vi "SimplePulseGenerator.vi"() -> ()   [LabVIEW 2012]
uses:
  <vilib>/Utility/sysdir.llb/System Directory Type.ctl
  <vilib>/Utility/miscctls.llb/LVPointTypeDef.ctl
  <vilib>/DAQmx/create/channels.llb/DAQmx Create Channel (CO-Pulse Generation-Frequency).vi
  <vilib>/DAQmx/configure/timing.llb/DAQmx Timing (Implicit).vi
  <resource>/objmgr/daqmx.rc
panel:
  out "title":string="Simple PulseGenerator"
  in  "Output Pulse Count":u64 caption="Pulse" format="%.0p"
  in  "Chk Finite":bool
  in  "Duty Cycle(%)":i32(slide)=50 scale=1.0..99.0
  in  "Counter Ch":tag="Dev1/ctr0"
  in  "Idle State":i32(ring)=10214 items=["High"=10192, "Low"=10214]
  in  "Frequency(Hz)":i32(knob)=1000 scale=1.0..1000000.0 scale format="%.0p"
  in  "Output":bool caption="Output Sw"
  # "with DAQmx Driver"
  # "%"
  # "Hz"
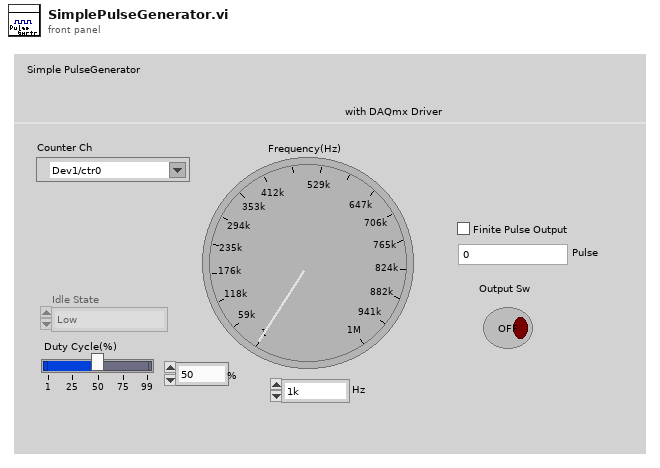
[diagram p1: front panel]
types:
  T1 = enum32{"invalid app kind", "Development System", "Run Time System", "Student Edition", "Embedded LabVIEW", "Evaluation", "Custom"}
  T2 = typedef "System Directory Type.ctl" = i32
  T3 = typedef "LVPointTypeDef.ctl" = cluster{"Horizontal":i16, "Vertical":i16}
  T4 = cluster{bool, "include Ctrl key?":bool, string}[]
  T5 = cluster{"配列[0]":i16, "配列[1]":i16, "配列[2]":i16, "配列[3]":i16}
  T6 = typedef "LVRectTypeDef.ctl" = cluster{"Left":i16, "Top":i16, "Right":i16, "Bottom":i16}
  T7 = enum8{"Enabled", "Disabled", "Disabled and Grayed Out"}
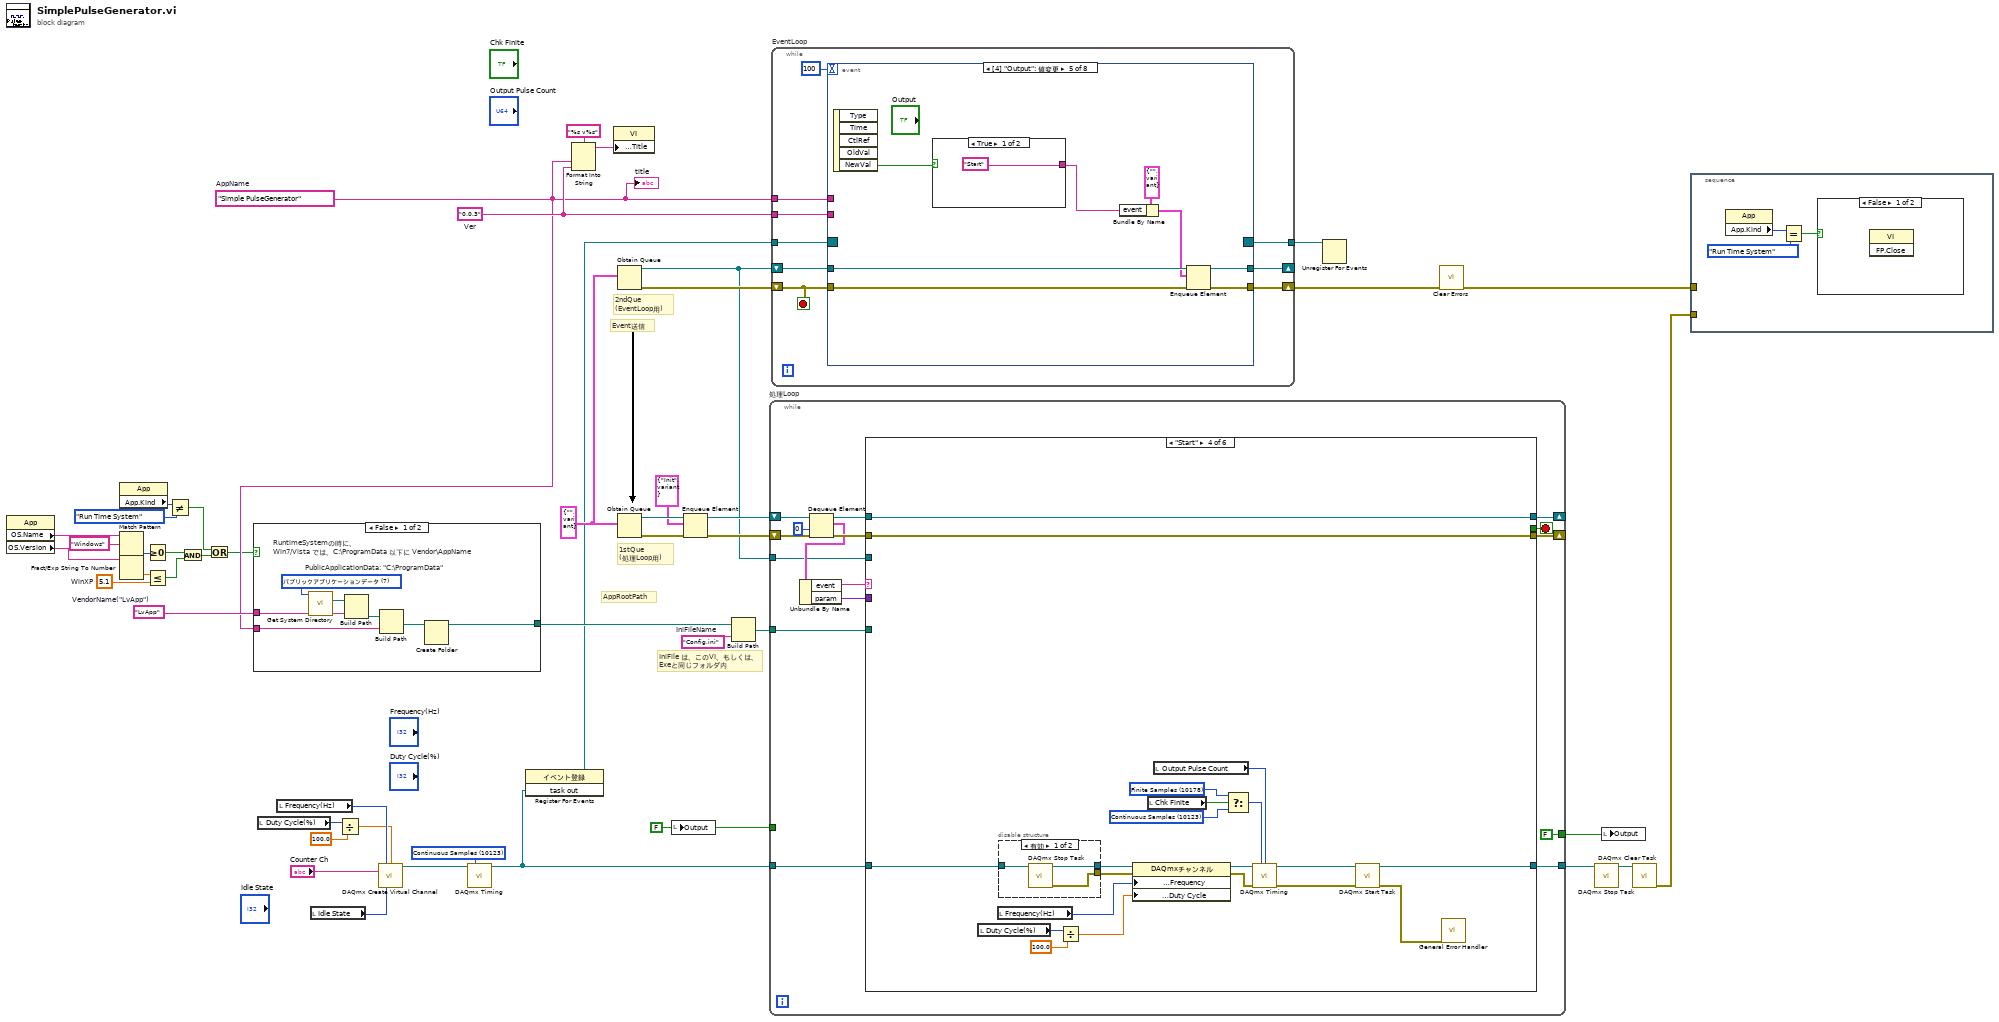
[diagram p0: block diagram]
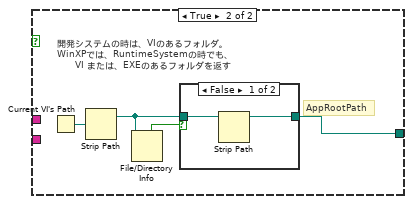
[diagram p2: hidden frame]
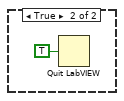
[diagram p4: hidden frame]
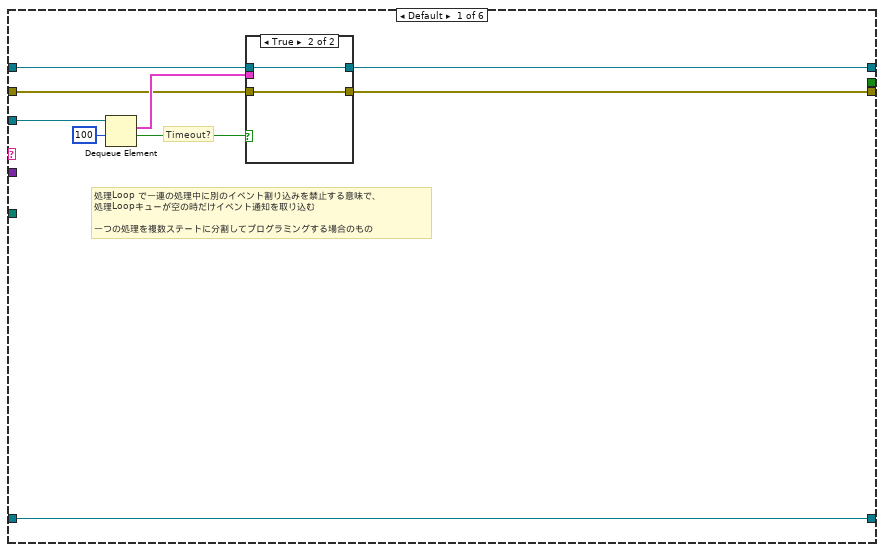
[diagram p5: hidden frame]
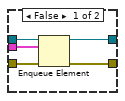
[diagram p6: hidden frame]
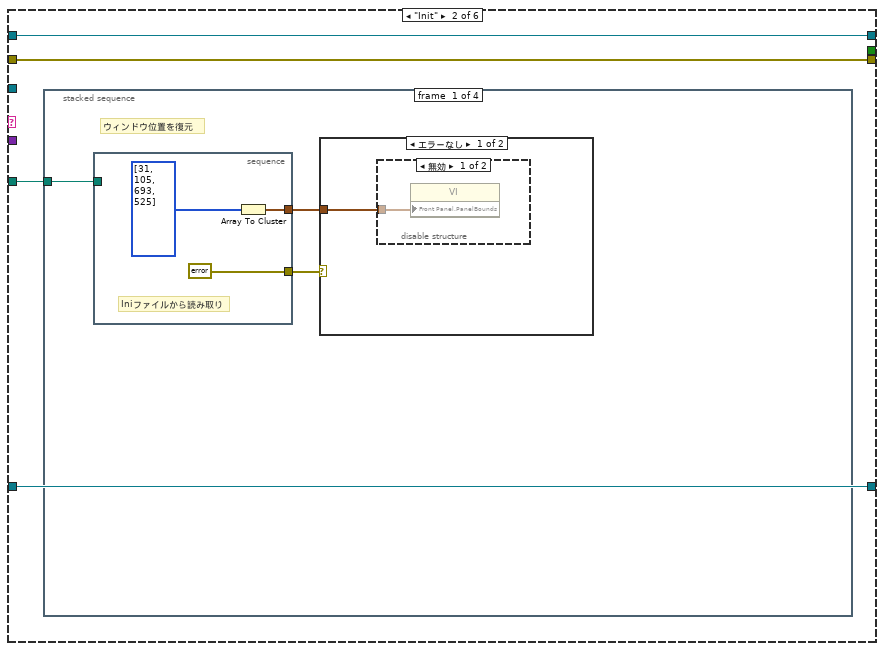
[diagram p7: hidden frame]
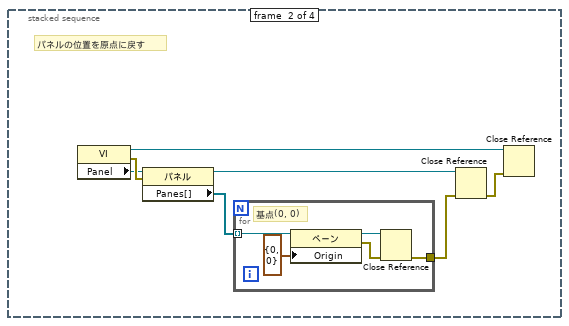
[diagram p10: hidden frame]
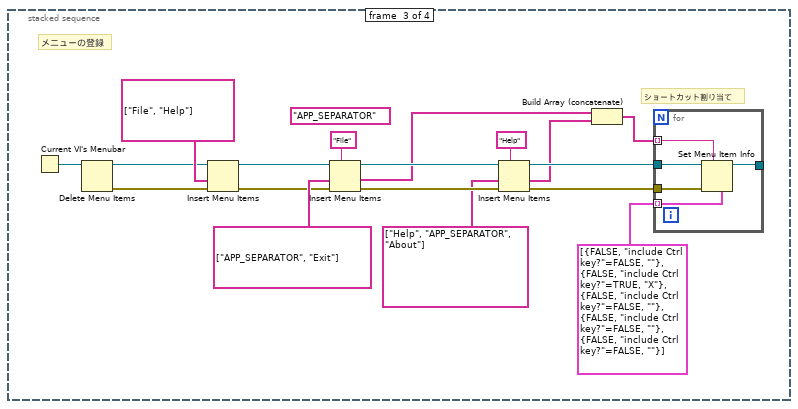
[diagram p11: hidden frame]
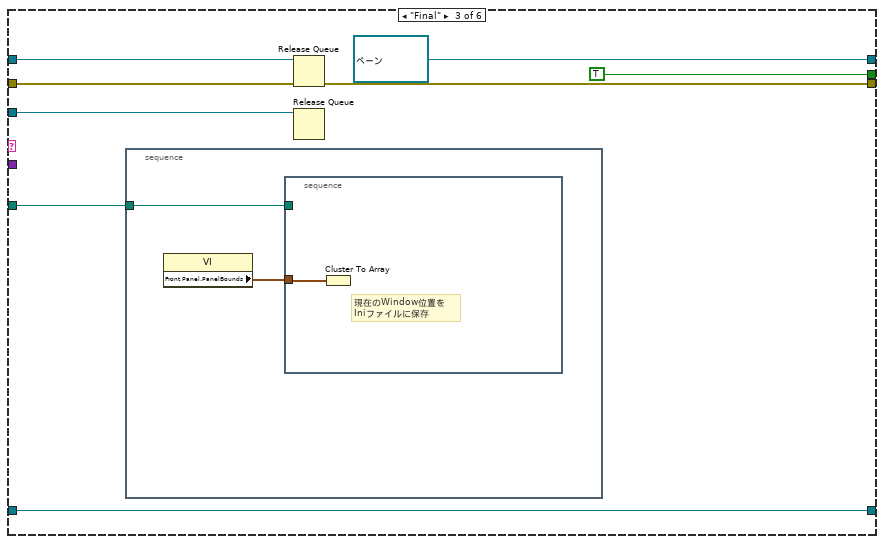
[diagram p13: hidden frame]
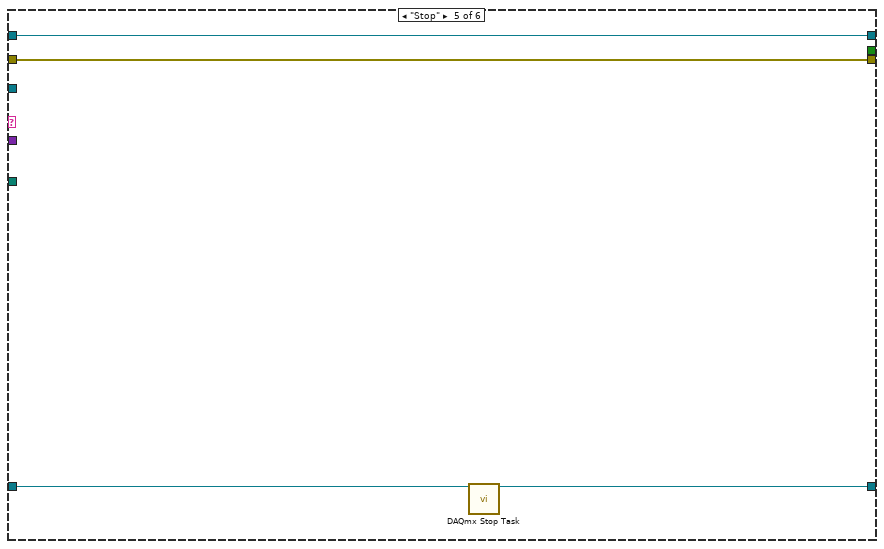
[diagram p15: hidden frame]
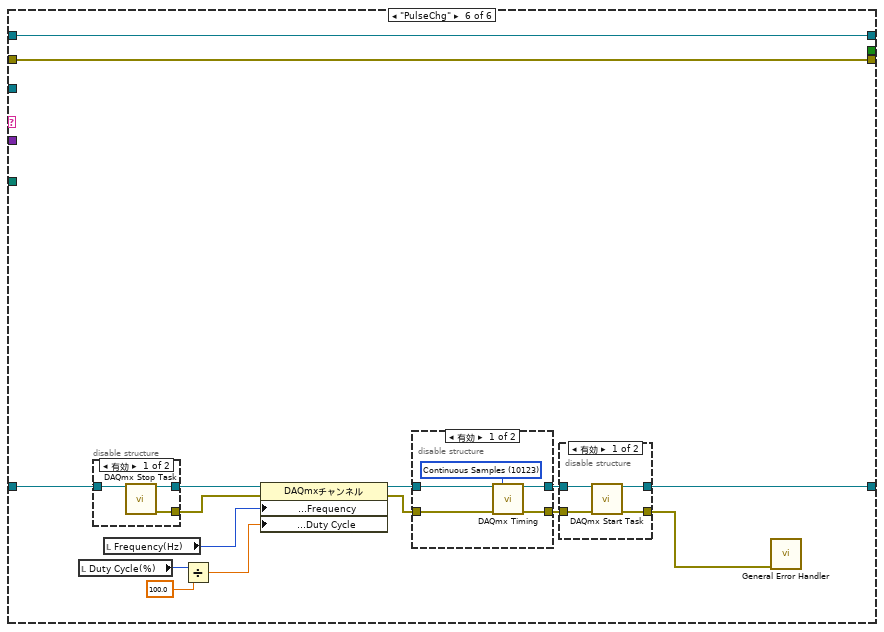
[diagram p16: hidden frame]
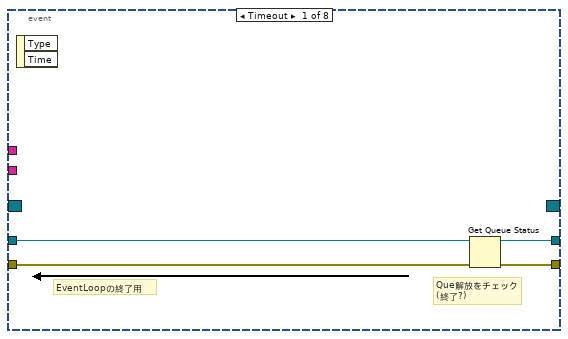
[diagram p20: hidden frame]
diagram:
  w6 = 10123 items=["Finite Samples"=10178, "Continuous Samples"=10123] ("sample mode")
  w12 = cluster{"event":string, "param":variant} {"event"="", "param"=variant}
  w14 = FALSE ("Output")
  w24 = "LvApp"  # VendorName("LvApp")
  w29 = 5.1  # WinXP
  w34 = "Config.ini"  # IniFileName
  w37 = "0.0.3"  # Ver
  w23 = "Simple PulseGenerator"  # AppName
  # "IniFile は、このVI、もしくは、\nExeと同じフォルダ内"
  # "AppRootPath"
  # "2ndQue\n(EventLoop用)"
  # "1stQue\n(処理Loop用)"
  # "Event送信"
  n1 = property class="App"() -> ("OS.Name"=w33:string, "OS.Version"=w31:string)  [unwired: 2 in, 2 out]
  n2 = Match Pattern(string=w33, regular expression="Windows" ("正規表現")) -> (offset past match=w28:i32)  [unwired: 1 in, 3 out]
  n3 = Fract/Exp String To Number(string=w31) -> (number=w30:dbl)  [unwired: 3 in, 1 out]
  n4 = property class="App"() -> ("App.Kind"=w22:T1)  [unwired: 2 in, 2 out]
  n5 = Greater Or Equal To 0?(x=w28) -> (x >= 0?=w27:bool)
  n6 = Less Or Equal?(x=w30, y=w29) -> (x <= y?=w26:bool)
  n7 = Not Equal?(x=w22, y=T1."Run Time System" ("アプリケーション:種類")) -> (x != y?=w20:bool)
  n8 = And(x=w27, y=w26) -> (x .and. y?=w19:bool)
  n9 = Or(x=w20, y=w19) -> (x .or. y?=w18:bool)
  n10 = case shown="FALSE" w18 {
    tunnel: w23 -> [w51 _]
    tunnel: [w48 w55] -> w25
    tunnel: w24 -> [w49 _]
    frame False {
      w54 = T2 7 items=["ユーザホーム"=0, "ユーザデスクトップ"=1, "ユーザドキュメント"=2, "ユーザアプリケーションデータ"=3, "ユーザ設定"=4, "ユーザ一時"=5, "パブリックドキュメント"=6, "パブリックアプリケーションデータ"=7, "パブリック環境設定"=8, "パブリックキャッシュ"=13, "システムコアライブラリ"=9, "システムインストールされたライブラリ"=10, "アプリケーションファイル"=11, "ブート容量ルート"=12] ("system directory type")
      # "RuntimeSystemの時に、\nWin7/Vista では、C:\\ProgramData 以下に Vendor\\AppName"
      # "PublicApplicationData: \"C:\\ProgramData\""
      n11 = call <vilib>:"Get System Directory.vi"("system directory type"=w54) -> ("system directory"=w53:path)  [unwired: 10 in]
      n12 = Build Path(base path=w53, name or relative path=w49) -> (appended path=w52:path)
      n13 = Build Path(base path=w52, name or relative path=w51) -> (appended path=w50:path)
      n14 = Create Folder(path (use dialog)=w50) -> (created path=w48:path)  [unwired: 2 in, 2 out]
    }
    frame True {
      # "開発システムの時は、VIのあるフォルダ。\nWinXPでは、RuntimeSystemの時でも、\n　　VI または、EXEのあるフォルダを返す"
      # "AppRootPath"
      n15 = Current VI's Path() -> (path=w58:path)
      n16 = Strip Path(path=w58) -> (stripped path=w57:path)  [unwired: 1 out]
      n17 = File/Directory Info(path=w57) -> (directory=w56:bool)  [unwired: 1 in, 6 out]
      n18 = case shown="FALSE" w56 {
        tunnel: w57 -> [w60 w61]
        tunnel: [w59 w61] -> w55
        frame False {
          n19 = Strip Path(path=w60) -> (stripped path=w59:path)  [unwired: 1 out]
        }
        frame True {
        }
      }
    }
  }
  n20 = local read "Duty Cycle(%)"() -> (w10:i32)
  n21 = local read "Frequency(Hz)"() -> (w8:i32)
  n22 = local read "Idle State"() -> (w16:i32)
  n23 = Divide(x=w10, y=100.0) -> (x/y=w7:dbl)
  n24 = call-poly <vilib>:"DAQmx Create Virtual Channel.vi"("frequency"=w8, "duty cycle"=w7, "counter"="Counter Ch", "idle state"=w16) -> ("task out"=w5:refnum<k21>)  [unwired: 10 in, 1 out]
  n25 = call-poly <vilib>:"DAQmx Timing.vi"("task/channels in"=w5, "sample mode"=w6) -> ("task out"=w3:refnum<k21>)  [unwired: 12 in, 1 out]
  n26 = register-events(w3) -> (reference out=w2:refnum<event-registration>)  [unwired: 2 in, 1 out]
  n27 = Format Into String(format string="%s v%s" ("形式文字列"), w23, w37) -> (resulting string=w35:string)  [unwired: 2 in, 1 out]
  n28 = property class="VI"("Front Panel.Title"=w35) -> ()  [unwired: 2 in, 2 out]
  n29 = Obtain Queue(element data type=w12) -> (queue out=w41:refnum<queue>, error out=w47:errorcluster)  [unwired: 4 in, 1 out]
  n30 = Obtain Queue(element data type=w12) -> (queue out=w46:refnum<queue>, error out=w44:errorcluster)  [unwired: 4 in, 1 out]
  n31 = local write "Output"(w14) -> ()
  n32 = Enqueue Element(queue=w46, element=cluster{string, "バリアント":variant} {"Init", "バリアント"=variant}, error in (no error)=w44) -> (queue out=w45:refnum<queue>, error out=w43:errorcluster)  [unwired: 1 in, 1 out]
  n33 = Build Path(base path=w25, name or relative path=w34) -> (appended path=w38:path)
  n34 = while "処理Loop" {
    shift-right: [w72] -> _
    shift-left: w45 -> [w77]
    shift-right: [w71] -> _
    shift-left: w43 -> [w74]
    tunnel: w41 -> [w67]
    tunnel: w38 -> [w65]
    tunnel: w3 -> [w64]
    tunnel: [w63] -> w15
    tunnel: w14 -> [_]
    tunnel: [FALSE] -> w11
    stop <- w66 stop-if-true
    n35 = Dequeue Element(queue=w77, timeout in ms (-1)=0 ("タイムアウト（ms）（-1）"), error in (no error)=w74) -> (queue out=w76:refnum<queue>, element=w70:cluster{"event":string, "param":variant}, error out=w73:errorcluster)  [unwired: 1 out]
    n36 = Unbundle By Name(w70) -> ("event"=w69:string, "param"=w68:variant)
    n37 = case shown="\"Start\"" w69 {
      tunnel: w76 -> [w83 w97 w147 w171 w179 w194]
      tunnel: w67 -> [w86 _ w145 _ _ _]
      tunnel: w73 -> [w81 w96 w144 w170 w178 w193]
      tunnel: [w82 w97 refnum<queue> refnum ("queue out") w171 w179 w194] -> w72
      tunnel: [w80 w96 w143 w170 w178 w193] -> w71
      tunnel: w68 -> [_ _ _ _ _ _]
      tunnel: [_ _ TRUE _ _ _] -> w66
      tunnel: w65 -> [_ w95 w142 _ _ _]
      tunnel: w64 -> [w78 w94 w141 w163 w177 w190]
      tunnel: [w78 w94 w141 w162 w176 w185] -> w63
      frame Default {
        # "Timeout?"
        # "処理Loop で一連の処理中に別のイベント割り込みを禁止する意味で、\n処理Loopキューが空の時だけイベント通知を取り込む\n\n一つの処理を複数ステートに分割してプログラミングする場合のもの"
        n38 = Dequeue Element(queue=w86, timeout in ms (-1)=100 ("タイムアウト（ms）（-1）")) -> (element=w84:cluster{"event":string, "param":variant}, timed out?=w79:bool)  [unwired: 1 in, 2 out]
        n39 = case shown="TRUE" w79 {
          tunnel: w84 -> [w91 _]
          tunnel: w83 -> [w90 w93]
          tunnel: [w89 w93] -> w82
          tunnel: w81 -> [w88 w92]
          tunnel: [w87 w92] -> w80
          frame False {
            n40 = Enqueue Element(queue=w90, element=w91, error in (no error)=w88) -> (queue out=w89:refnum<queue>, error out=w87:errorcluster)  [unwired: 1 in, 1 out]
          }
          frame True {
          }
        }
      }
      frame "Init" {
        n41 = stacked-sequence {
          tunnel: w95 -> [w98 _ _ _]
          frame #0 {
            # "ウィンドウ位置を復元"
            n42 = stacked-sequence {
              tunnel: [w101] -> w100
              tunnel: [errorcluster {"status"=FALSE, "code"=0, "source"=""} ("error in (no error)")] -> w99
              tunnel: w98 -> [_]
              frame #0 {
                # "Iniファイルから読み取り"
                n43 = Array To Cluster(array=i16[] [31, 105, 693, 525] ("配列")) -> (cluster=w101:T5)
              }
            }
            n44 = case shown="エラーなし" w99 {
              tunnel: w100 -> [w104 _]
              frame No Error {
                n45 = disable-structure shown="無効" {
                  disable-tunnel: w104 -> [w105 _]
                  frame Disabled {
                    n46 = property class="VI"("Front Panel.PanelBounds"=w105) -> ()  [unwired: 2 in, 2 out]
                  }
                  frame Enabled {
                  }
                }
              }
              frame Error {
              }
            }
          }
          frame #1 {
            # "パネルの位置を原点に戻す"
            n47 = property class="VI"() -> (reference out=w109:refnum<vi>, error out=w112:errorcluster, "Panel"=w106:refnum<vi>)  [unwired: 2 in]
            n48 = property on="プロパティノード" class="パネル"(reference=w106, error in=w112) -> (reference out=w108:refnum<vi>, "Panes[]"=w107:refnum<vi>[])  [unwired: 1 out]
            n49 = for {
              tunnel: w107 -> [w117] mode=indexing
              tunnel: [w114] -> w110
              # "基点(0, 0)"
              n50 = property on="プロパティノード" class="ペーン"(reference=w117, "Origin"=T3 {"Horizontal"=0, "Vertical"=0} ("原点")) -> (reference out=w116:refnum<vi>, error out=w115:errorcluster)  [unwired: 1 in]
              n51 = Close Reference(reference=w116, error in (no error)=w115) -> (error out=w114:errorcluster)
            }
            n52 = Close Reference(reference=w108, error in (no error)=w110) -> (error out=w111:errorcluster)
            n53 = Close Reference(reference=w109, error in (no error)=w111) -> ()  [unwired: 1 out]
          }
          frame #2 {
            (unwired) "APP_SEPARATOR"
            # "ショートカット割り当て"
            # "メニューの登録"
            n54 = Current VI's Menubar() -> (w126:refnum<k9>)
            n55 = Delete Menu Items(9:w126) -> (0:w128:errorcluster, 3:w127:refnum<k9>)  [unwired: 3 in]
            n56 = Insert Menu Items(6:w128, 7:string[] ["File", "Help"] ("item tags"), 9:w127) -> (0:w132:errorcluster, 3:w131:refnum<k9>)  [unwired: 3 in, 1 out]
            n57 = Insert Menu Items(5:"File" ("menu tag"), 6:w132, 7:string[] ["APP_SEPARATOR", "Exit"] ("item tags"), 9:w131) -> (0:w135:errorcluster, 1:w121:string[], 3:w134:refnum<k9>)  [unwired: 2 in]
            n58 = Insert Menu Items(5:"Help" ("menu tag"), 6:w135, 7:string[] ["Help", "APP_SEPARATOR", "About"] ("item tags"), 9:w134) -> (0:w122:errorcluster, 1:w120:string[], 3:w123:refnum<k9>)  [unwired: 2 in]
            n59 = Build Array (concatenate)(w121, w120) -> (w118:string[])
            n60 = for {
              tunnel: w123 -> [w140]
              tunnel: w122 -> [w139]
              tunnel: [w138] -> _
              tunnel: T4 [{FALSE, "include Ctrl key?"=FALSE, ""}, {FALSE, "include Ctrl key?"=TRUE, "X"}, {FALSE, "include Ctrl key?"=FALSE, ""}, {FALSE, "include Ctrl key?"=FALSE, ""}, {FALSE, "include Ctrl key?"=FALSE, ""}] -> [w137] mode=indexing
              tunnel: w118 -> [w136] mode=indexing
              n61 = Set Menu Item Info(4:w137, 7:w136, 8:w139, 11:w140) -> (3:w138:refnum<k9>)  [unwired: 3 in, 1 out]
            }
          }
          frame #3 {
            # "パネル制御器の初期化"
          }
        }
      }
      frame "Final" {
        n62 = stacked-sequence {
          tunnel: w142 -> [w150]
          frame #0 {
            n63 = property class="VI"() -> ("Front Panel.PanelBounds"=w149:T6)  [unwired: 2 in, 2 out]
            n64 = stacked-sequence {
              tunnel: w150 -> [_]
              tunnel: w149 -> [w151]
              frame #0 {
                # "現在のWindow位置を\nIniファイルに保存"
                n65 = Cluster To Array(cluster=w151) -> ()  [unwired: 1 out]
              }
            }
          }
        }
        n66 = Release Queue(queue=w147, error in (no error)=w144) -> (error out=w143:errorcluster)  [unwired: 1 in, 2 out]
        n67 = Release Queue(queue=w145) -> ()  [unwired: 2 in, 3 out]
      }
      frame "Start" {
        w155 = 10178 items=["Finite Samples"=10178, "Continuous Samples"=10123] ("sample mode")
        w154 = 10123 items=["Finite Samples"=10178, "Continuous Samples"=10123] ("sample mode")
        n68 = local read "Duty Cycle(%)"() -> (w159:i32)
        n69 = local read "Frequency(Hz)"() -> (w158:i32)
        n70 = disable-structure shown="有効" {
          disable-tunnel: [w174 w175] -> w167
          disable-tunnel: [w173 _] -> w166
          disable-tunnel: w163 -> [w172 w175]
          frame Enabled {
            n71 = call <vilib>:"DAQmx Stop Task.vi"("task/channels in"=w172) -> ("task out"=w174:refnum<k21>, "error out"=w173:errorcluster)  [unwired: 13 in]
          }
          frame Disabled {
          }
        }
        n72 = Divide(x=w159, y=100.0) -> (x/y=w157:dbl)
        n73 = property class="DAQmxチャンネル"(reference=w167, error in=w166, "Counter Output:Pulse:Frequency:Frequency"=w158, "Counter Output:Pulse:Frequency:Duty Cycle"=w157) -> (reference out=w168:refnum<k21>, error out=w169:errorcluster)
        n74 = local read "Chk Finite"() -> (w156:bool)
        n75 = local read "Output Pulse Count"() -> (w152:u64)
        n76 = Select(t=w155, s=w156, f=w154) -> (s? t:f=w153:i32)
        n77 = call-poly <vilib>:"DAQmx Timing.vi"("task/channels in"=w168, "sample mode"=w153, "samples per channel"=w152, "error in"=w169) -> ("task out"=w165:refnum<k21>, "error out"=w164:errorcluster)  [unwired: 10 in]
        n78 = call <vilib>:"DAQmx Start Task.vi"("task/channels in"=w165, "error in"=w164) -> ("task out"=w162:refnum<k21>, "error out"=w161:errorcluster)  [unwired: 12 in]
        n79 = call <vilib>:"General Error Handler.vi"("error in (no error)"=w161) -> ()  [unwired: 10 in, 5 out]
      }
      frame "Stop" {
        n80 = call <vilib>:"DAQmx Stop Task.vi"("task/channels in"=w177) -> ("task out"=w176:refnum<k21>)  [unwired: 13 in, 1 out]
      }
      frame "PulseChg" {
        n81 = local read "Duty Cycle(%)"() -> (w182:i32)
        n82 = disable-structure shown="有効" {
          disable-tunnel: w190 -> [w210 w211]
          disable-tunnel: [w209 w211] -> w189
          disable-tunnel: [w208 _] -> w188
          frame Enabled {
            n83 = call <vilib>:"DAQmx Stop Task.vi"("task/channels in"=w210) -> ("task out"=w209:refnum<k21>, "error out"=w208:errorcluster)  [unwired: 13 in]
          }
          frame Disabled {
          }
        }
        n84 = local read "Frequency(Hz)"() -> (w181:i32)
        n85 = Divide(x=w182, y=100.0) -> (x/y=w180:dbl)
        n86 = property class="DAQmxチャンネル"(reference=w189, error in=w188, "Counter Output:Pulse:Frequency:Frequency"=w181, "Counter Output:Pulse:Frequency:Duty Cycle"=w180) -> (reference out=w191:refnum<k21>, error out=w192:errorcluster)
        n87 = disable-structure shown="有効" {
          disable-tunnel: w192 -> [w199 w200]
          disable-tunnel: w191 -> [w198 w201]
          disable-tunnel: [w196 w201] -> w187
          disable-tunnel: [w195 w200] -> w186
          frame Enabled {
            w197 = 10123 items=["Finite Samples"=10178, "Continuous Samples"=10123] ("sample mode")
            n88 = call-poly <vilib>:"DAQmx Timing.vi"("task/channels in"=w198, "sample mode"=w197, "error in"=w199) -> ("task out"=w196:refnum<k21>, "error out"=w195:errorcluster)  [unwired: 11 in]
          }
          frame Disabled {
          }
        }
        n89 = disable-structure shown="有効" {
          disable-tunnel: w187 -> [w205 w207]
          disable-tunnel: w186 -> [w204 w206]
          disable-tunnel: [w203 w207] -> w185
          disable-tunnel: [w202 w206] -> w184
          frame Enabled {
            n90 = call <vilib>:"DAQmx Start Task.vi"("task/channels in"=w205, "error in"=w204) -> ("task out"=w203:refnum<k21>, "error out"=w202:errorcluster)  [unwired: 12 in]
          }
          frame Disabled {
          }
        }
        n91 = call <vilib>:"General Error Handler.vi"("error in (no error)"=w184) -> ()  [unwired: 10 in, 5 out]
      }
    }
  }
  n92 = while "EventLoop" {
    shift-right: [w218] -> _
    shift-left: w41 -> [w219]
    shift-right: [w217] -> w40
    shift-left: w47 -> [w216]
    tunnel: w23 -> [w215]
    tunnel: w37 -> [w214]
    tunnel: w2 -> [w213]
    tunnel: [w212] -> w1
    stop <- w216 stop-if-true
    n93 = event shown="[4] \"Output\": 値変更" {
      selector: w213 -> [_ _ _ _ _ _ _ _]
      dyn-events: [_ _ _ _ _ _ _ _] -> w212
      timeout: 100 -> [_ _ _ _ _ _ _ _]
      tunnel: w219 -> [w224 w230 w238 w253 w276 w286 w291 w306]
      tunnel: [w221 w229 w237 w252 w275 w285 w290 w306] -> w218
      tunnel: w216 -> [w223 w228 w236 w251 w274 w284 w289 w305]
      tunnel: [w222 w227 w235 w250 w273 w283 w288 w305] -> w217
      tunnel: w215 -> [_ _ _ w248 _ _ _ _]
      tunnel: w214 -> [_ _ _ w247 _ _ _ _]
      event Timeout {
        # "EventLoopの終了用"
        # "Que解放をチェック\n(終了?)"
        n94 = event-data() -> ()  [unwired: 1 in, 2 out]
        n95 = Get Queue Status(queue=w224, error in (no error)=w223) -> (queue out=w221:refnum<queue>, error out=w222:errorcluster)  [unwired: 1 in, 6 out]
      }
      event Application Instance Close? {
        n96 = event-data() -> ()  [unwired: 1 in, 4 out]
        n97 = Enqueue Element(queue=w230, element=cluster{string, "バリアント":variant} {"Final", "バリアント"=variant}, error in (no error)=w228) -> (queue out=w229:refnum<queue>, error out=w227:errorcluster)  [unwired: 1 in, 1 out]
        n98 = event-data("SilentShutdown"=TRUE, "Discard?"=FALSE ("破棄?")) -> ()  [unwired: 1 in, 1 out]
      }
      event Panel Close? {
        n99 = event-data() -> ()  [unwired: 1 in, 3 out]
        n100 = Two Button Dialog(message="App Exit?" ("メッセージ"), 2:"Exit" ("Tボタン名（\"OK\"）")) -> (T button?=w234:bool)  [unwired: 1 in]
        n101 = case shown="FALSE" w234 {
          tunnel: w238 -> [w240 w246]
          tunnel: [w240 w245] -> w237
          tunnel: w236 -> [w241 w244]
          tunnel: [w241 w243] -> w235
          frame False {
          }
          frame True {
            n102 = Enqueue Element(queue=w246, element=cluster{string, "バリアント":variant} {"Final", "バリアント"=variant}, error in (no error)=w244) -> (queue out=w245:refnum<queue>, error out=w243:errorcluster)  [unwired: 1 in, 1 out]
          }
        }
        n103 = event-data("Discard?"=TRUE) -> ()  [unwired: 1 in, 1 out]
      }
      event Menu Selection (User) {
        n104 = event-data() -> ("ItemPath"=w249:string)  [unwired: 1 in, 5 out]
        n105 = case shown="\"Help:About\"" w249 {
          tunnel: w253 -> [w255 w260 w266 w268]
          tunnel: [w255 w259 w266 w268] -> w252
          tunnel: w251 -> [w254 w258 w265 w267]
          tunnel: [w254 w257 w265 w267] -> w250
          tunnel: w248 -> [_ _ w264 _]
          tunnel: w247 -> [_ _ w263 _]
          frame Default {
          }
          frame "File:Exit" {
            n106 = Enqueue Element(queue=w260, element=cluster{string, "バリアント":variant} {"Final", "バリアント"=variant}, error in (no error)=w258) -> (queue out=w259:refnum<queue>, error out=w257:errorcluster)  [unwired: 1 in, 1 out]
          }
          frame "Help:About" {
            n107 = Format Into String(format string="%s\n\nVersion : %s" ("メッセージ"), w264, w263) -> (resulting string=w261:string)  [unwired: 2 in, 1 out]
            n108 = One Button Dialog(message=w261) -> ()  [unwired: 1 in, 1 out]
          }
          frame "Help:Help" {
          }
        }
      }
      event "Output": Value Change {
        n109 = event-data() -> ("NewVal"=w272:bool)  [unwired: 1 in, 4 out]
        n110 = case shown="TRUE" w272 {
          tunnel: ["Start" ("event") "Stop" ("event")] -> w269
          frame True {
          }
          frame False {
          }
        }
        n111 = Bundle By Name(cluster=cluster{"event":string, "param":variant} {"event"="", "param"=variant}, "event"=w269) -> (w270:cluster{"event":string, "param":variant})
        n112 = Enqueue Element(queue=w276, element=w270, error in (no error)=w274) -> (queue out=w275:refnum<queue>, error out=w273:errorcluster)  [unwired: 1 in, 1 out]
      }
      event Done {
        n113 = event-data() -> ()  [unwired: 1 in, 5 out]
        n114 = local write "Output"(FALSE ("Output")) -> ()
        n115 = Bundle By Name(cluster=cluster{"event":string, "param":variant} {"event"="", "param"=variant}, "event"="Stop") -> (w281:cluster{"event":string, "param":variant})
        n116 = Enqueue Element(queue=w286, element=w281, error in (no error)=w284) -> (queue out=w285:refnum<queue>, error out=w283:errorcluster)  [unwired: 1 in, 1 out]
      }
      event "Frequency(Hz)", "Duty Cycle(%)": Value Change {
        n117 = event-data() -> ()  [unwired: 1 in, 5 out]
        n118 = local read "Output"() -> (w287:bool)
        n119 = case shown="TRUE" w287 {
          tunnel: w291 -> [w293 w300]
          tunnel: [w293 w299] -> w290
          tunnel: w289 -> [w292 w298]
          tunnel: [w292 w297] -> w288
          frame False {
          }
          frame True {
            n120 = Bundle By Name(cluster=cluster{"event":string, "param":variant} {"event"="", "param"=variant}, "event"="PulseChg") -> (w295:cluster{"event":string, "param":variant})
            n121 = Enqueue Element(queue=w300, element=w295, error in (no error)=w298) -> (queue out=w299:refnum<queue>, error out=w297:errorcluster)  [unwired: 1 in, 1 out]
          }
        }
      }
      event "Chk Finite": Value Change {
        n122 = event-data() -> ("NewVal"=w304:bool)  [unwired: 1 in, 4 out]
        n123 = Select(t=T7."Enabled" ("無効"), s=w304, f=T7."Disabled and Grayed Out" ("無効")) -> (s? t:f=w303:T7)
        n124 = property on="Output Pulse Count" class="DigNum （指定）"("DisabledEnum"=w303) -> ()  [unwired: 2 in, 2 out]
      }
    }
  }
  n125 = Unregister For Events(event registration refnum=w1) -> ()  [unwired: 1 in, 1 out]
  n126 = call <vilib>:"Clear Errors.vi"("error in (no error)"=w40) -> ("error out"=w39:errorcluster)  [unwired: 6 in]
  n127 = call <vilib>:"DAQmx Stop Task.vi"("task/channels in"=w15) -> ("task out"=w13:refnum<k21>)  [unwired: 13 in, 1 out]
  n128 = local write "Output"(w11) -> ()
  n129 = call <vilib>:"DAQmx Clear Task.vi"("task in"=w13) -> ("error out"=w4:errorcluster)  [unwired: 14 in]
  n130 = stacked-sequence {
    tunnel: w39 -> [_]
    tunnel: w4 -> [_]
    frame #0 {
      n131 = property class="App"() -> ("App.Kind"=w309:T1)  [unwired: 2 in, 2 out]
      n132 = Equal?(x=w309, y=T1."Run Time System" ("アプリケーション:種類")) -> (x = y?=w307:bool)
      n133 = case shown="FALSE" w307 {
        frame False {
          n134 = invoke class="VI" method="FP.Close"() -> ()  [unwired: 3 in, 3 out]
        }
        frame True {
          n135 = Quit LabVIEW(quit? (T)=TRUE ("終了?（T）")) -> ()
        }
      }
    }
  }
  "title" <- w23
